vi "Remove All Shields.vi"(8 "error in (no error)":errorcluster, 9 "Packed refs":T1, 10 "Board Game in":refnum<class "Board Game.lvclass">, 11 "Shield in":refnum<class "Shield.lvclass">) -> (0 "error out":errorcluster, 3 "Shield out":refnum<class "Shield.lvclass">)   [LabVIEW 2021, in "Shield.lvclass"]
uses:
  Shield.lvclass
  C:/Users/poche/Programs/LabVIEW/imposible snake/GameEl_class/GameEl.lvclass
  Board Game_class/Board Game.lvclass
  Application/Packed Refs.ctl
  GameEl_class/private/Enum Direction.ctl
  Imposible_Snake_v2/LVApp/Modules/Sound Manager/Typedefs/Sound Effects.ctl
  GameEl_class/GameEl.lvclass/GameEl.ctl
  Shield.lvclass/Shield.ctl
  Board Game_class/Board Game.lvclass/Board Game.ctl
  Board Game_class/Read Shield Ref.vi
  GameEl_class/GameEl.lvclass
  Imposible_Snake_v2/LVApp/Modules/Sound Manager/Sound Manager.lvlib
  Application/Game.lvclass
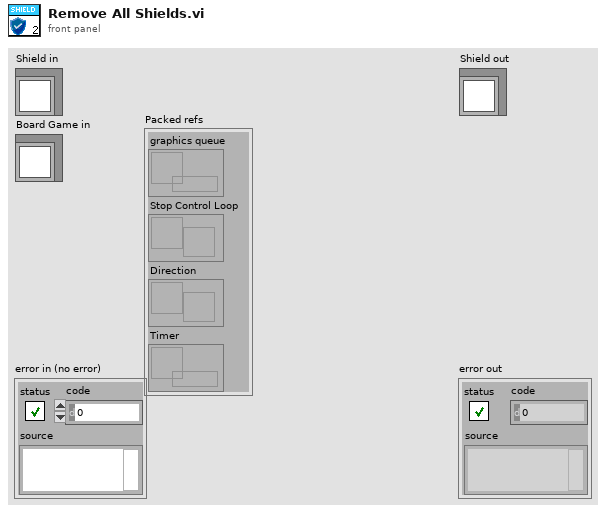
[diagram p1: front panel]
types:
  T1 = typedef "Game.lvclass/Packed Refs.ctl" = cluster{"graphics queue":refnum<queue>, "Stop Control Loop":refnum<user-event>, "Direction":refnum<notifier>, "Timer":refnum<data-value>}
  T2 = typedef "Sound Manager.lvlib/Sound Effects.ctl" = enum16{"Bomb In", "Bomb Out", "Bomb Touched", "Game Over", "Victory", "Eat", "10 Fruits", "Eat2", "Eat3", "Eat4", "MaxShield", "Shield", "10p", "Grape In", "Grape Out", "20p", "30p", "40p", "50p", "60p", "70p", "80p", "90p", "100p", "All shields cracked", "Mouse In", "Mouse Out", "Mouse Eaten", "Grape Eaten", "States Recover", "Broken Shield", "Bonus", "Happy Time", "explode", "Game over musica", "Back Music", "Shield Catch", "Evil lough", "Cricket In", "Cricket eaten", "Lets Go", "Jump1", "Jump2", "Jump3", "Unstoppable", "Troll Music", "winner", "menu"}
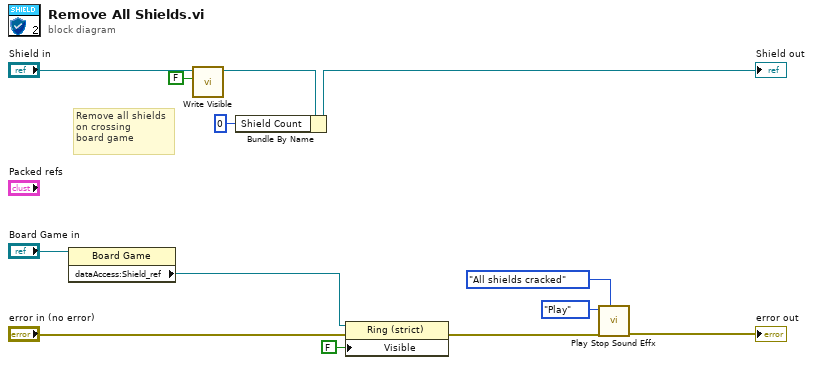
[diagram p0: block diagram]
diagram:
  # "Remove all shields\non crossing \nboard game"
  n1 = property class="Board Game"(reference="Board Game in") -> ("dataAccess:Shield_ref"=w6:refnum<vi>)  [unwired: 1 in, 2 out]
  n2 = call "Write Visible.vi"("Visible"=FALSE, "GameEl in"="Shield in") -> ("GameEl out"=w12:refnum<class "Shield.lvclass">)  [unwired: 8 in, 1 out]
  n3 = Bundle By Name(cluster=w12, "Shield Count"=u8 0) -> (→"Shield out":refnum<class "Shield.lvclass">)
  n4 = property class="Ring (strict)"(reference=w6, error in="error in (no error)", "Visible"=FALSE) -> (error out=w2:errorcluster)  [unwired: 1 out]
  n5 = call "Play Stop Sound Effx.vi"("Sound Effect"=Sound_Effects."All shields cracked", "Error In"=w2, "Function"=enum16{"Play", "Stop"}."Play") -> ("error in (no error)"=→"error out":errorcluster)  [unwired: 8 in]
